vi "GetSystemDefinitionPropertyValue_String.vi"(8 "error in (no error)":errorcluster, 10 "property name":string, 11 "BaseNodeType in":refnum<k24>) -> (0 "error out":errorcluster, 2 "value":string, 3 "BaseNodeType out":refnum<k24>)   [LabVIEW 2015, in "VeriStandTestUtilities.lvlib"]
uses:
  VeriStandTestUtilities.lvlib
  NationalInstruments.VeriStand.SystemStorage
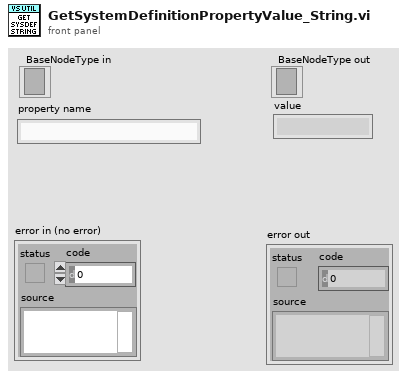
[diagram p1: front panel]
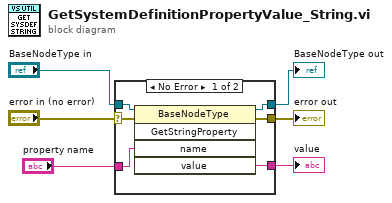
[diagram p0: block diagram]
diagram:
  n1 = case shown="No Error" "error in (no error)" {
    selector: "error in (no error)" -> [w11 w14]
    tunnel: "BaseNodeType in" -> [w12 w13]
    tunnel: "property name" -> [w10 _]
    tunnel: [w9 w13] -> w3
    tunnel: [w8 w14] -> w2
    tunnel: [w7 _] -> w1
    frame No Error {
      n2 = invoke class="BaseNodeType" method="GetStringProperty"(reference=w12, error in=w11, "name"=w10) -> (reference out=w9:refnum<k24>, error out=w8:errorcluster, "value"=w7:string)  [unwired: 2 in, 2 out]
    }
    frame Error {
    }
  }
  "error out" <- w2
  "BaseNodeType out" <- w3
  "value" <- w1
